vi "API String to 1D Array.vi"(8 "SEPERATOR":enum16{"0x2C - ,", "0x3B - ;"}(ring), 9 "TYPE":T1(ring), 10 "string":string) -> (2 "Array of Strings":string[](array[string])=["sin(x)+2", "VIA(x", "y)", " VIB(z)"])   [LabVIEW 2017]
uses:
  <userlib>/_NEVSTOP/Communicable State Machine(CSM)/Communicable State Machine.lvlib
  API-String-Arugments-Support/API String Arguments Support.lvlib
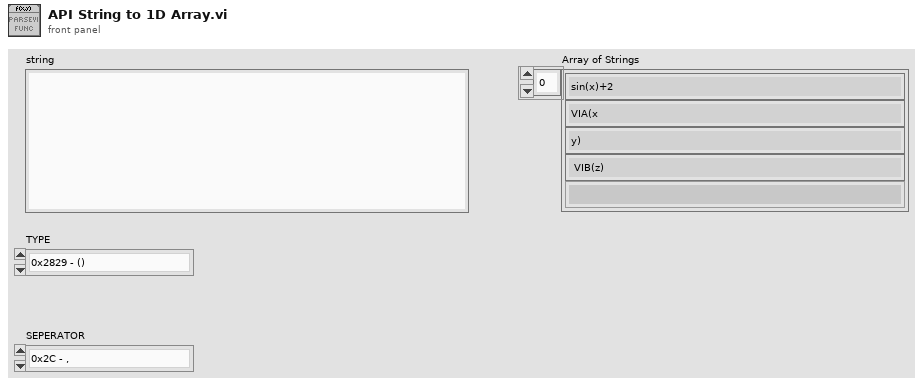
[diagram p1: front panel]
types:
  T1 = enum16{"0x2829 - ()", "0x5B5D - []", "0x7B7D - {}"}
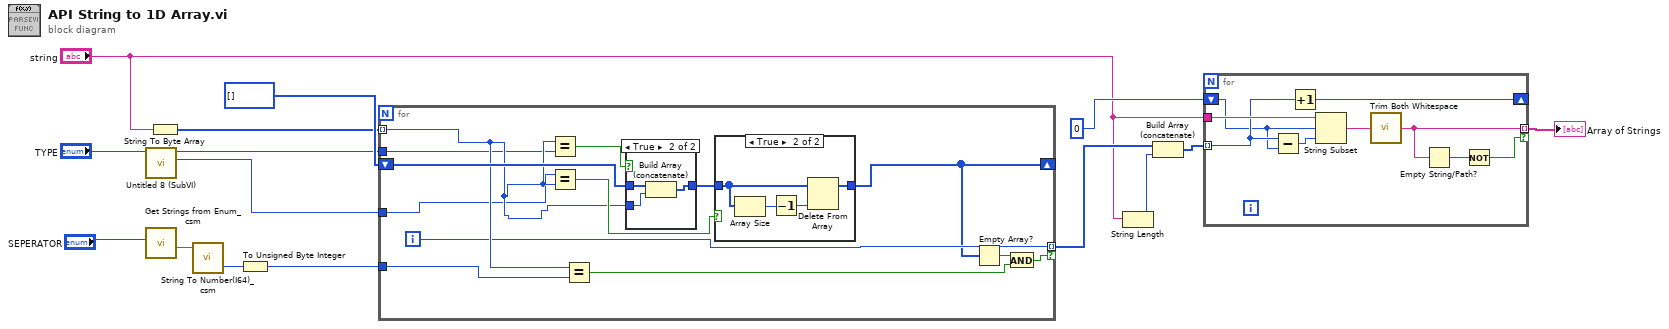
[diagram p0: block diagram]
diagram:
  n1 = call "Untitled 8 (SubVI).vi"("Enum"="TYPE") -> ("Numeric"=w6:u8, "Numeric 2"=w7:u8)  [unwired: 9 in]
  n2 = call <userlib>:"Get Strings from Enum_csm.vi"("Enum"="SEPERATOR") -> ("String Value"=w5:string)  [unwired: 7 in, 3 out]
  n3 = String To Byte Array(string="string") -> (unsigned byte array=w14:u8[])
  n4 = call "String To Number(I64)_csm.vi"("String"=w5) -> ("Numeric(I64)"=w3:u64)  [unwired: 4 in]
  n5 = To Unsigned Byte Integer(number=w3) -> (unsigned 8bit integer=w2:u8)
  n6 = for {
    tunnel: w14 -> [w24] mode=indexing
    shift-right: [w21] -> _
    shift-left: i32[] [] -> [w25]
    tunnel: [w23] -> w13 mode=indexing if=w20
    tunnel: w7 -> [w18]
    tunnel: w6 -> [w17]
    tunnel: w2 -> [w16]
    i -> [w23]
    n7 = Equal?(x=w24, y=w18) -> (x = y?=w28:bool)
    n8 = Equal?(x=w17, y=w24) -> (x = y?=w26:bool)
    n9 = Equal?(x=w24, y=w16) -> (x = y?=w19:bool)
    n10 = case shown="True" w28 {
      tunnel: w25 -> [w34 w37]
      tunnel: w24 -> [_ w36]
      tunnel: [w34 w35] -> w27
      frame False {
      }
      frame True {
        n11 = Build Array (concatenate)(w37, w36) -> (w35:i32[])
      }
    }
    n12 = case shown="True" w26 {
      tunnel: w27 -> [w29 w32]
      tunnel: [w29 w30] -> w21
      frame False {
      }
      frame True {
        n13 = Array Size(array=w32) -> (size(s)=w33:i32)
        n14 = Decrement(x=w33) -> (x-1=w31:i32)
        n15 = Delete From Array(array=w32, index=w31) -> (array with subset deleted=w30:i32[])  [unwired: 1 in, 1 out]
      }
    }
    n16 = Empty Array?(array=w21) -> (empty?=w22:bool)
    n17 = And(x=w22, y=w19) -> (x .and. y?=w20:bool)
  }
  n18 = String Length(string="string") -> (length=w9:i32)
  n19 = Build Array (concatenate)(w13, w9) -> (w10:i32[])
  n20 = for {
    tunnel: "string" -> [w46]
    tunnel: w10 -> [w44] mode=indexing
    tunnel: [w40] -> w11 mode=indexing if=w38
    shift-right: [w41] -> _
    shift-left: 0 ("Numeric") -> [w42]
    n21 = Subtract(x=w44, y=w42) -> (x-y=w43:i32)
    n22 = Increment(x=w44) -> (x+1=w41:i32)
    n23 = String Subset(string=w46, offset (0)=w42, length (rest)=w43) -> (substring=w45:string)
    n24 = call <userlib>:"Trim Both Whitespace.vi"("string"=w45) -> ("trimmed string"=w40:string)  [unwired: 1 in]
    n25 = Empty String/Path?(string/path=w40) -> (empty?=w39:bool)
    n26 = Not(x=w39) -> (.not. x?=w38:bool)
  }
  "Array of Strings" <- w11
